vi "Debug.vi"(4 "Numeric 1":dbl=nan, 6 "Numeric 0":dbl=nan, 8 "error in (no error)":errorcluster, 9 "Numeric 3":dbl=nan, 10 "Numeric 2":dbl=nan, 11 "Stepper in":refnum<class "Stepper.lvclass">) -> (0 "error out":errorcluster, 3 "Stepper out":refnum<class "Stepper.lvclass">)   [LabVIEW 2015, in "Stepper.lvclass"]
uses:
  Stepper.lvclass
  CO2 Actor/CO2 Actor.lvclass
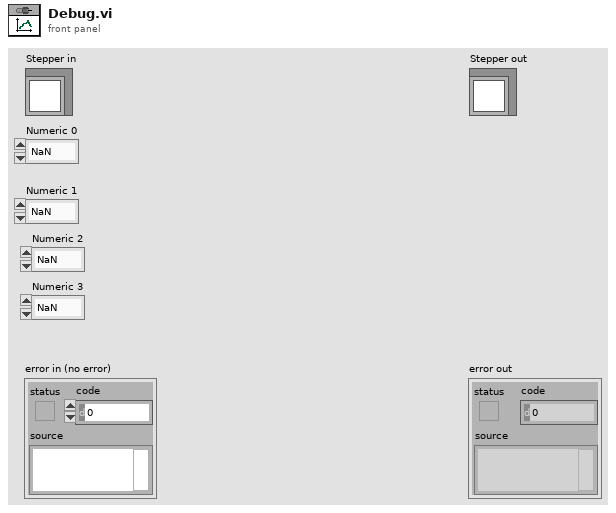
[diagram p1: front panel]
types:
  T1 = cluster{"Numeric 0":dbl, "Numeric 1":dbl, "Numeric 2":dbl, "Numeric 3":dbl, "Numeric 4":dbl, "Numeric 5":dbl, "Numeric 6":dbl, "Numeric 7":dbl}
  T2 = typedef "cRIO-Carbondioxide.lvlib/cRIO-CO2.lvlib/cRIO-CO2.lvclass/Debugger.ctl" = cluster{"Log Ref":refnum<vi>, "Debugger Graph Chart Ref":refnum<vi>, "Debug Rng Ref":refnum<vi>}
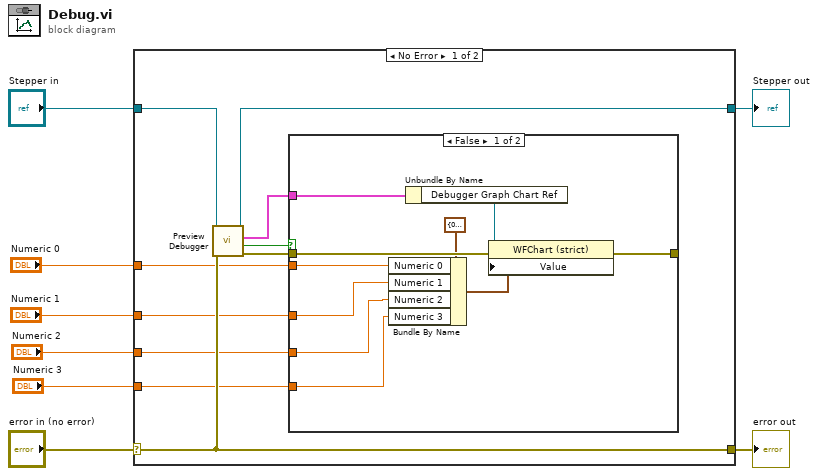
[diagram p0: block diagram]
diagram:
  n1 = case shown="No Error" "error in (no error)" {
    selector: "error in (no error)" -> [w18 w30]
    tunnel: [w18 w30] -> w7
    tunnel: [w15 w29] -> w5
    tunnel: "Stepper in" -> [w16 w29]
    tunnel: "Numeric 0" -> [w12 _]
    tunnel: "Numeric 1" -> [w11 _]
    tunnel: "Numeric 2" -> [w10 _]
    tunnel: "Numeric 3" -> [w9 _]
    frame No Error {
      n2 = call "Preview Debugger.vi"("error in (no error)"=w18, "CO2 Actor in"=w16) -> ("error out"=w13:errorcluster, "timed out?"=w14:bool, "Debugger"=w17:T2, "CO2 Actor out"=w15:refnum<class "Stepper.lvclass">)  [unwired: 6 in]
      n3 = case shown="False" w14 {
        tunnel: w17 -> [w28 _]
        tunnel: w13 -> [w26 _]
        tunnel: w12 -> [w23 _]
        tunnel: [w22 _] -> _
        tunnel: w11 -> [w21 _]
        tunnel: w10 -> [w20 _]
        tunnel: w9 -> [w19 _]
        frame False {
          n4 = Bundle By Name(cluster=T1 {"Numeric 0"=0.0, "Numeric 1"=nan, "Numeric 2"=nan, "Numeric 3"=nan, "Numeric 4"=nan, "Numeric 5"=nan, "Numeric 6"=nan, "Numeric 7"=nan} ("Debugger Graph Chart"), "Numeric 0"=w23, "Numeric 1"=w21, "Numeric 2"=w20, "Numeric 3"=w19) -> (w24:T1)
          n5 = Unbundle By Name(w28) -> ("Debugger Graph Chart Ref"=w27:refnum<vi>)
          n6 = property class="WFChart (strict)"(reference=w27, error in=w26, "Value"=w24) -> (error out=w22:errorcluster)  [unwired: 1 out]
        }
        frame True {
        }
      }
    }
    frame Error {
    }
  }
  "error out" <- w7
  "Stepper out" <- w5
